vi "FlexDDS-NG_USB_VISA_Open.vi"(11 "FlexDDS-NG USB VISA resource name (COM)":refnum<visa-resource-name>="COM5") -> (0 "error out":errorcluster, 3 "FlexDDS-NG USB VISA resource name out":refnum<visa-resource-name>)   [LabVIEW 2016]
uses:
  <vilib>/Instr/_visa.llb/VISA Configure Serial Port (Instr).vi
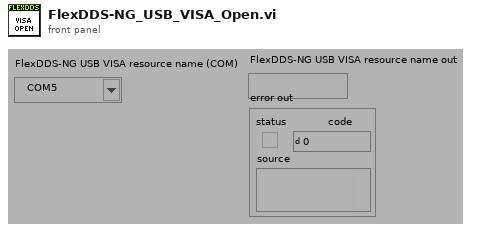
[diagram p1: front panel]
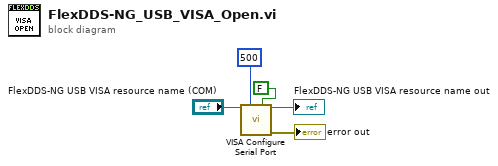
[diagram p0: block diagram]
diagram:
  n1 = call-poly "VISA Configure Serial Port"("VISA resource name"="FlexDDS-NG USB VISA resource name (COM)", "timeout (10sec)"=u32 500, "Enable Termination\nChar (T)"=FALSE ("Enable Termination\nChar (T)")) -> ("VISA resource name out"=→"FlexDDS-NG USB VISA resource name out":refnum<visa-resource-name>, "error out"=→"error out":errorcluster)  [unwired: 11 in]
